vi "g2_4fold_g4.vi"() -> ()   [LabVIEW 2020]
uses:
  <vilib>/Math Plots/2D Math Plots/2D Error Bar/2D Error Bar XCtrl/2D Error Bar.xctl
  C:/Program Files/Dotfast Consulting/Timetag Explorer 2.26/ttInterface.dll
  Program Files/Dotfast Consulting/Timetag Explorer 2.26/ttInterface.dll
  <vilib>/Utility/file.llb/Write Delimited Spreadsheet (string).vi
  <vilib>/Utility/file.llb/Write Delimited Spreadsheet (I64).vi
  <vilib>/Math Plots/2D Math Plots/2D Error Bar/2D Error Bar Datatype/Public/Plot Helper (Fixed).vi
  <vilib>/Math Plots/2D Math Plots/2D Error Bar/2D Error Bar Datatype/2D Error Bar Datatype.lvclass
  <vilib>/Analysis/NI_AALBase.lvlib
panel:
  in  "#StepsR":i32
  out "S1_S2":refnum<class "2D Plot Datatype.lvclass">[](xcontrol)
  out "Intensity Graph":dbl[][](graph)
  out "R1vsR2iter":i32
  out "appended array":i32[](array[numeric])
  out "R2_S1_S2":refnum<class "2D Plot Datatype.lvclass">[](xcontrol)
  out "S1vsS2iter":i32
  in  "Acq Time (s)":dbl=0.1 format="%#_13g"
  out "R1_R2_S1_S2":refnum<class "2D Plot Datatype.lvclass">[](xcontrol)
  in  "# StepsS":i32
  in  "stop":bool
  in  "fileName":string
  in  "Folder":path
  in  "CTW in ns":dbl
  out "GetTimeCounter":i32
  out "GetResolution":dbl
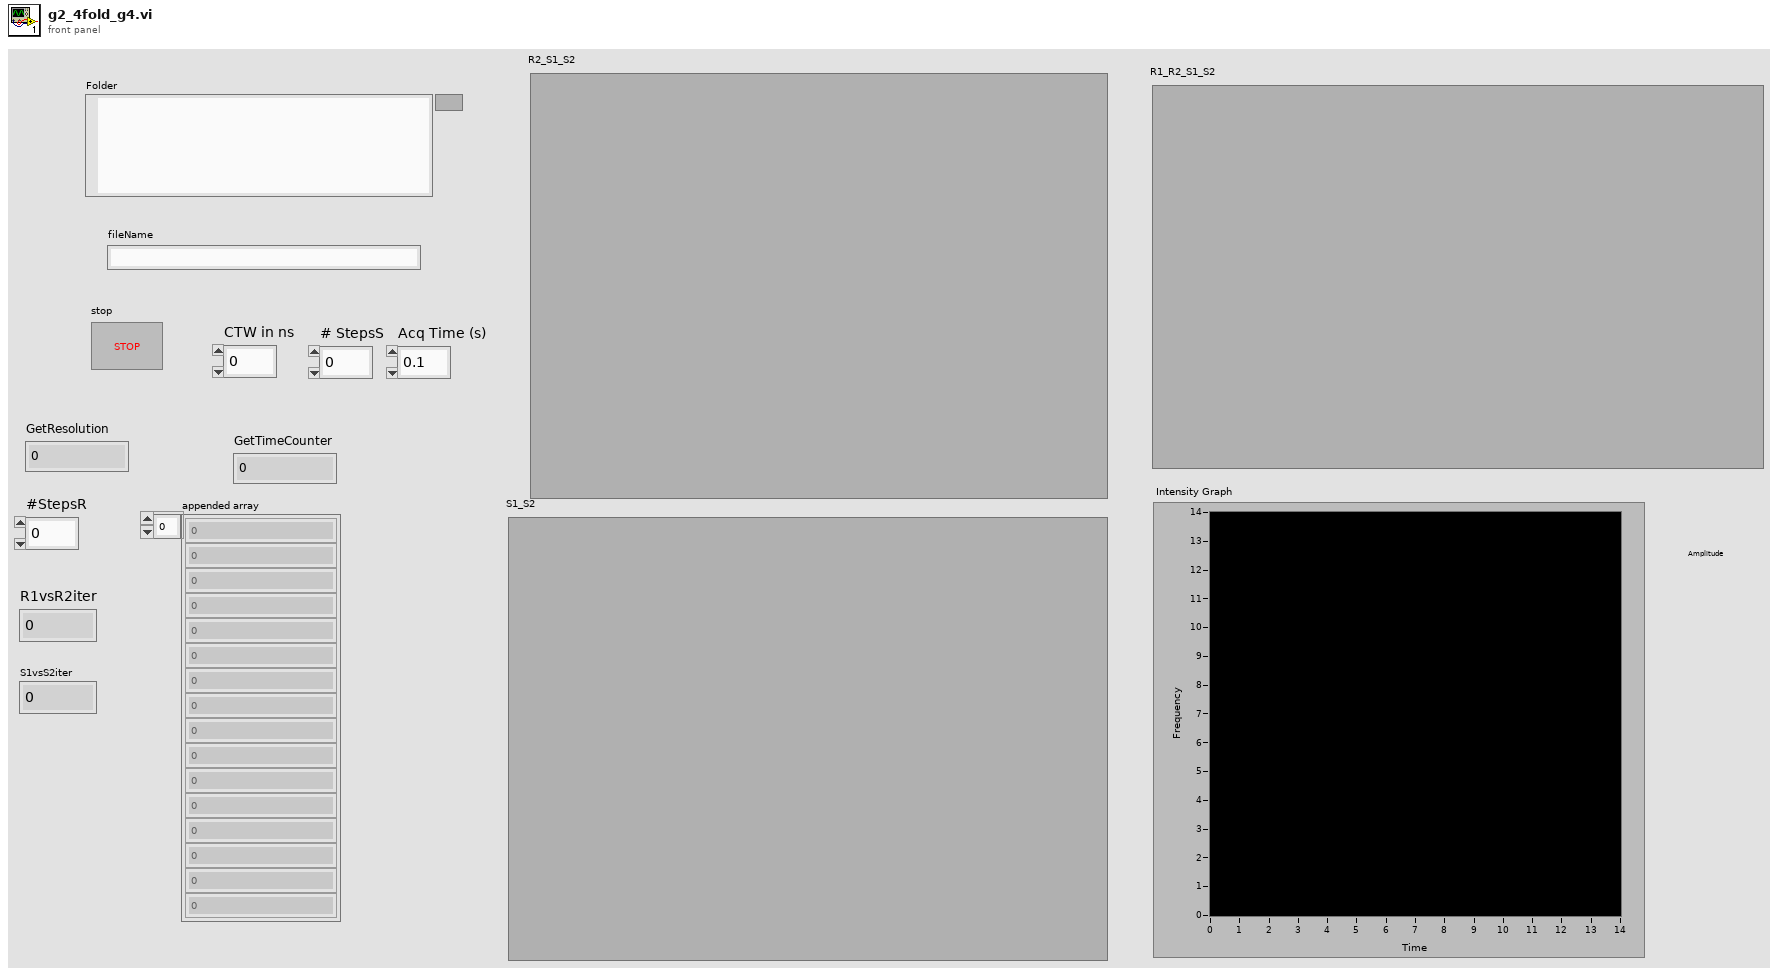
[diagram p1: front panel]
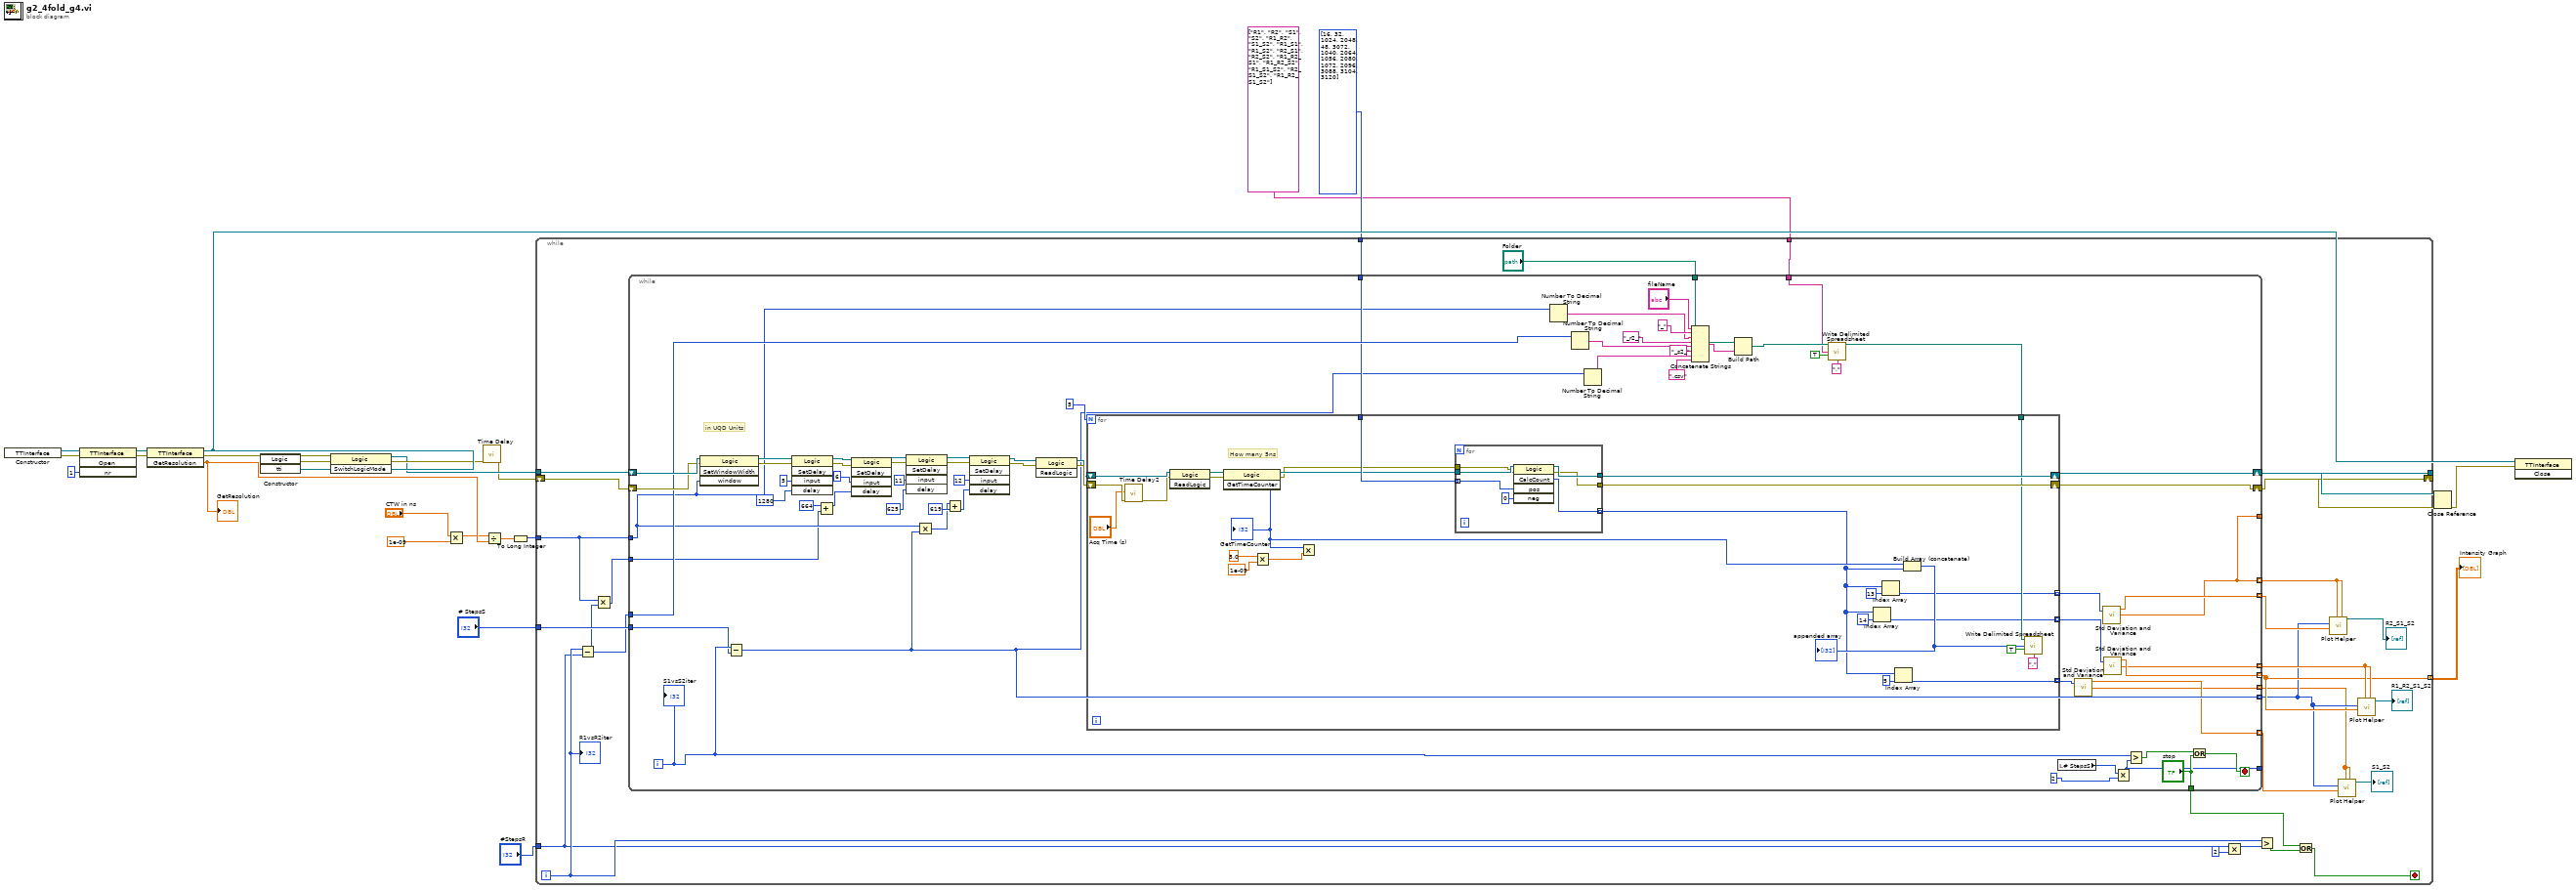
[diagram p0: block diagram]
diagram:
  n1 = constructor class="TTInterface"() -> (reference out=w26:refnum<k24>, error out=w25:errorcluster)  [unwired: 3 in, 1 out]
  n2 = invoke class="TTInterface" method="Open"(reference=w26, error in=w25, "nr"=1) -> (reference out=w22:refnum<k24>, error out=w23:errorcluster)  [unwired: 1 in, 2 out]
  n3 = invoke class="TTInterface" method="GetResolution"(reference=w22, error in=w23) -> (reference out=w21:refnum<k24>, error out=w20:errorcluster, "GetResolution"=w14:dbl)  [unwired: 1 in]
  "GetResolution" <- w14
  n4 = constructor class="Logic"(error in=w20, "tti"=w21) -> (reference out=w19:refnum<k24>, error out=w18:errorcluster)  [unwired: 2 in, 2 out]
  n5 = invoke class="Logic" method="SwitchLogicMode"(reference=w19, error in=w18) -> (reference out=w16:refnum<k24>, error out=w17:errorcluster)  [unwired: 1 in, 1 out]
  n6 = Multiply(x="CTW in ns", y=1e-09) -> (x*y=w13:dbl)
  n7 = call "Time Delay"("error in (no error)"=w17) -> ("error out"=w15:errorcluster)  [unwired: 10 in]
  n8 = Divide(x=w13, y=w14) -> (x/y=w12:dbl)
  n9 = To Long Integer(number=w12) -> (32bit integer=w9:i32)
  n10 = while {
    tunnel: w16 -> [w54]
    tunnel: w9 -> [w40]
    tunnel: "# StepsS" -> [w41]
    shift-right: [w50] -> w6
    shift-left: w15 -> [w53]
    tunnel: [w51] -> w8
    tunnel: i32[] [16, 32, 1024, 2048, 48, 3072, 1040, 2064, 1056, 2080, 1072, 2096, 3088, 3104, 3120] -> [w37]
    tunnel: string[] ["R1", "R2", "S1", "S2", "R1_R2", "S1_S2", "R1_S1", "R1_S2", "R2_S1", "R2_S2", "R1_R2_S1", "R1_R2_S2", "R1_S1_S2", "R2_S1_S2", "R1_R2_S1_S2"] -> [w36]
    tunnel: [w35] -> w2 mode=indexing
    tunnel: "#StepsR" -> [w33]
    i -> [w42]
    stop <- w43 stop-if-true
    n11 = Subtract(x=w42, y=w33) -> (x-y=w34:i32)
    n12 = Multiply(x=w40, y=w34) -> (x*y=w39:i32)
    n13 = while {
      shift-right: [w97] -> w51
      shift-left: w54 -> [w116]
      shift-right: [w96] -> w50
      shift-left: w53 -> [w115]
      tunnel: "Folder" -> [w112]
      tunnel: w40 -> [w64]
      tunnel: w41 -> [w100]
      tunnel: [w95] -> w46 mode=indexing
      tunnel: [w81] -> w38 mode=indexing
      tunnel: [w65] -> w28 mode=indexing
      tunnel: [w94] -> w35 mode=indexing
      tunnel: [w93] -> w47 mode=indexing
      tunnel: ["stop"] -> w45
      tunnel: [w86] -> _
      tunnel: w39 -> [w60]
      tunnel: w34 -> [w82]
      tunnel: [w81] -> _
      tunnel: w37 -> [w80]
      tunnel: w36 -> [w76]
      tunnel: [w56] -> w29 mode=indexing
      tunnel: [w55] -> w27 mode=indexing
      i -> [w101]
      stop <- w110 stop-if-true
      # "in UQD Units"
      n14 = invoke class="Logic" method="SetWindowWidth"(reference=w116, error in=w115, "window"=w64) -> (reference out=w114:refnum<k24>, error out=w113:errorcluster)  [unwired: 1 in, 2 out]
      n15 = Subtract(x=w101, y=w100) -> (x-y=w65:i32)
      n16 = invoke class="Logic" method="SetDelay"(reference=w114, error in=w113, "input"=5, "delay"=1280) -> (reference out=w74:refnum<k24>, error out=w73:errorcluster)  [unwired: 1 in, 3 out]
      n17 = Add(x=664 ("delay"), y=w60) -> (x+y=w61:i32)
      n18 = invoke class="Logic" method="SetDelay"(reference=w74, error in=w73, "input"=6, "delay"=w61) -> (reference out=w72:refnum<k24>, error out=w71:errorcluster)  [unwired: 1 in, 3 out]
      n19 = invoke class="Logic" method="SetDelay"(reference=w72, error in=w71, "input"=11, "delay"=625) -> (reference out=w108:refnum<k24>, error out=w107:errorcluster)  [unwired: 1 in, 3 out]
      n20 = Multiply(x=w64, y=w65) -> (x*y=w62:i32)
      n21 = Add(x=w62, y=619 ("delay")) -> (x+y=w63:i32)
      n22 = invoke class="Logic" method="SetDelay"(reference=w108, error in=w107, "input"=12, "delay"=w63) -> (reference out=w106:refnum<k24>, error out=w105:errorcluster)  [unwired: 1 in, 3 out]
      n23 = invoke class="Logic" method="ReadLogic"(reference=w106, error in=w105) -> (reference out=w118:refnum<k24>, error out=w119:errorcluster)  [unwired: 1 in, 1 out]
      n24 = Number To Decimal String(number=w64) -> (decimal integer string=w90:string)  [unwired: 1 in]
      n25 = Number To Decimal String(number=w82) -> (decimal integer string=w88:string)  [unwired: 1 in]
      n26 = Number To Decimal String(number=w65) -> (decimal integer string=w84:string)  [unwired: 1 in]
      n27 = Concatenate Strings("fileName", "_" ("string"), w90, "_r2_" ("string"), w88, "_s2_" ("string"), w84, ".csv" ("string")) -> (w111:string)
      n28 = Build Path(base path=w112, name or relative path=w111) -> (appended path=w77:path)
      n29 = call-poly <vilib>:"Write Delimited Spreadsheet.vi"("file path (dialog if empty)"=w77, "1D data"=w76, "append to file? (new file:F)"=TRUE, "delimiter (\\t)"="," ("delimiter (\\t)")) -> ("new file path (Not A Path if cancelled)"=w75:path)  [unwired: 10 in, 1 out]
      n30 = for {
        N: 5 -> [_]
        shift-right: [w130] -> w96
        shift-left: w119 -> [w145]
        shift-right: [w131] -> w97
        shift-left: w118 -> [w144]
        tunnel: w80 -> [w133]
        tunnel: w75 -> [w127]
        tunnel: [w125] -> w59 mode=indexing
        tunnel: [w123] -> w58 mode=indexing
        tunnel: [w120] -> w57 mode=indexing
        # "How many 5ns"
        n31 = call "Time Delay2"("error in (no error)"=w145, "Delay Time (s)"="Acq Time (s)") -> ("error out"=w143:errorcluster)  [unwired: 9 in]
        n32 = invoke class="Logic" method="ReadLogic"(reference=w144, error in=w143) -> (reference out=w138:refnum<k24>, error out=w137:errorcluster)  [unwired: 1 in, 1 out]
        n33 = invoke class="Logic" method="GetTimeCounter"(reference=w138, error in=w137) -> (reference out=w132:refnum<k24>, error out=w129:errorcluster, "GetTimeCounter"=w134:i32)  [unwired: 1 in]
        "GetTimeCounter" <- w134
        n34 = Multiply(x=5.0, y=1e-09) -> (x*y=w139:dbl)
        n35 = Multiply(x=w134, y=w139) -> ()  [unwired: 1 out]
        n36 = for {
          tunnel: w133 -> [w152] mode=indexing
          tunnel: w132 -> [w151]
          tunnel: [w149] -> w131
          tunnel: [w148] -> w130
          tunnel: w129 -> [w147]
          tunnel: [w146] -> w122 mode=indexing
          n37 = invoke class="Logic" method="CalcCount"(reference=w151, error in=w147, "pos"=w152, "neg"=0) -> (reference out=w149:refnum<k24>, error out=w148:errorcluster, "CalcCount"=w146:i32)  [unwired: 1 in, 2 out]
        }
        n38 = Index Array(array=w122, index=14) -> (element=w123:i32)
        n39 = Index Array(array=w122, index=13) -> (element=w125:i32)
        n40 = Index Array(array=w122, index=5) -> (element=w120:i32)
        n41 = Build Array (concatenate)(w134, w122) -> (w128:i32[])
        "appended array" <- w128
        n42 = call-poly <vilib>:"Write Delimited Spreadsheet.vi"("file path (dialog if empty)"=w127, "1D data"=w128, "append to file? (new file:F)"=TRUE, "delimiter (\\t)"="," ("delimiter (\\t)")) -> ()  [unwired: 10 in, 2 out]
      }
      n43 = local read "# StepsS"() -> (w99:i32)
      n44 = call <vilib>:"Std Deviation and Variance.vi"("X"=w57) -> ("mean"=w56:dbl, "standard deviation"=w55:dbl)  [unwired: 1 in, 1 out]
      n45 = call <vilib>:"Std Deviation and Variance.vi"("X"=w59) -> ("mean"=w95:dbl, "standard deviation"=w81:dbl)  [unwired: 1 in, 1 out]
      n46 = call <vilib>:"Std Deviation and Variance.vi"("X"=w58) -> ("mean"=w94:dbl, "standard deviation"=w93:dbl)  [unwired: 1 in, 1 out]
      n47 = Multiply(x=w99, y=2) -> (x*y=w86:i32)
      n48 = Greater?(x=w101, y=w86) -> (0:w109:bool)
      n49 = Or(x=w109, y="stop") -> (x .or. y?=w110:bool)
      "S1vsS2iter" <- w101
    }
    n50 = Multiply(x=w33, y=2) -> (x*y=w32:i32)
    n51 = Greater?(x=w42, y=w32) -> (0:w44:bool)
    n52 = Or(x=w45, y=w44) -> (x .or. y?=w43:bool)
    n53 = call-poly <vilib>:"Plot Helper.vi"("error b vector"=w38, "error a vector"=w38, "y vector"=w46, "x vector"=w28) -> ("2D Plot Class Obj Array out"=→"R2_S1_S2":refnum<class "2D Plot Datatype.lvclass">[])  [unwired: 2 in, 5 out]
    n54 = call-poly <vilib>:"Plot Helper.vi"("error b vector"=w27, "error a vector"=w27, "y vector"=w29, "x vector"=w28) -> ("2D Plot Class Obj Array out"=→"S1_S2":refnum<class "2D Plot Datatype.lvclass">[])  [unwired: 2 in, 5 out]
    n55 = call-poly <vilib>:"Plot Helper.vi"("error b vector"=w47, "error a vector"=w47, "y vector"=w35, "x vector"=w28) -> ("2D Plot Class Obj Array out"=→"R1_R2_S1_S2":refnum<class "2D Plot Datatype.lvclass">[])  [unwired: 2 in, 5 out]
    "R1vsR2iter" <- w42
  }
  "Intensity Graph" <- w2
  n56 = Close Reference(reference=w8, error in (no error)=w6) -> (error out=w7:errorcluster)
  n57 = invoke class="TTInterface" method="Close"(reference=w21, error in=w7) -> ()  [unwired: 1 in, 3 out]
